vi "0 OCU - Networked.vi"() -> ()   [LabVIEW 2011]
doc: "This is the current implementation of the operator control unit (OCU) for small RC boat controlled by a host computer. The following features are currently implemented:\n- override control of the rudden angle and sail value by control interface or using keys\n- ability to add missions before and during a run\n- indicators for all relevant system status information\n\nAuthor: Jared Kirschner"
uses:
  2-Think/2 Typedefs/setpoints to boat.ctl
  2-Think/2 Typedefs/sail setpt.ctl
  2-Think/2 Typedefs/rudder angle.ctl
  2-Think/2 Typedefs/Velocity.ctl
  2-Think/2 Typedefs/apparent wind direction.ctl
  2-Think/2 Typedefs/apparent wind speed.ctl
  2-Think/2 Typedefs/apparent wind.ctl
  2-Think/2 Typedefs/heading.ctl
  2-Think/2 Typedefs/UTM Location.ctl
  2-Think/2 Typedefs/Which Boat.ctl
  2-Think/2 Typedefs/generalized sensor status.ctl
  2-Think/2 Typedefs/indicator LED.ctl
  2-Think/2 Typedefs/generalized actuator status.ctl
  0x2-OCU-Think Comm/0x2 Typedefs/Waypoints List.ctl
  0x2-OCU-Think Comm/0x2 Typedefs/ocuWaypoint.ctl
  0x2-OCU-Think Comm/0x2 Typedefs/waypointTypes.ctl
  0x2-OCU-Think Comm/0x2 Typedefs/Current Waypoint.ctl
  2-Think/2 Typedefs/robot velocity.ctl
  0x2-OCU-Think Comm/0x2 Typedefs/manual override.ctl
  0x2-OCU-Think Comm/0x2 Typedefs/ocuMessage.ctl
  0x2-OCU-Think Comm/0x2 Typedefs/ocuCommands.ctl
  2-Think/2 Typedefs/eStopCommand.ctl
  0x2-OCU-Think Comm/0x2 Typedefs/RIO-OCU update controls.ctl
  2-Think/2 Typedefs/rate of turn.ctl
  2-Think/2 Typedefs/pitch and roll.ctl
  2-Think/2 Typedefs/absolute wind direction.ctl
  2-Think/2 Typedefs/absolute wind speed.ctl
  2-Think/2 Typedefs/absolute water current vector.ctl
  0x2-OCU-Think Comm/0x2 Classes/NetworkStreams/Reader/readType.ctl
  2-Think/2 Globals/2 Global.vi
  0x2-OCU-Think Comm/0x2 Classes/NetworkStreams/Reader/NetworkStreamReader.lvclass
  0x2-OCU-Think Comm/0x2 Classes/NetworkStreams/Writer/NetworkStreamWriter.lvclass
panel:
  out "Rudder Position":dbl(knob) scale=50.0..-50.0 scale format="%#.2g"
  out "Sail Position":dbl(knob)
  out "Last update":timestamp
  out "Connected?":bool caption="Connection Status"
  in  "Location of THINK":string(combo)="127.0.0.1"
  in  "OVERRIDE SAIL?":bool
  in  "OVERRIDE RUDDER?":bool
  in  "E-Stop":bool
  out "Override Rudder Angle":dbl(slide) scale=-50.0..50.0
  out "Override Sail Value":dbl(slide) scale=0.0..1.0
  in  "OCU Tab Control":T1(tab)=enum."Before Mission: Define Mission"
  out "Connected":bool
  in  "Connect":bool
  out "Rudder Actuator Status":T2
  out "Sail Actuator Status":T2
  out "Wind Sensor Status":T4
  in  "Map Path (relative)":path=path "locations/LPB Pool.png"
  out "# of Waypts":i32
  in  "Save Waypoints\nand PoI":bool
  in  "Save Image":bool
  out "Mission Map":T5(plugin-control)
  in  "Delete Last Waypoint":bool
  in  "Mission Def Filepath":path caption="MDF (Mission Definition File) path (leave blank for nothing)"
  in  "Next Point Dist/Time":dbl=0.5
  in  "Next Point Type":T6
  in  "Globals":T7(tab)
  out "Which Boat Am I?":T8
  out "Battery Voltage":dbl
  out "Robot Heading":T9 format="%05.1f"
  out "Robot UTM Location":T10
  out "Overview Image":T5(plugin-control)
  out "Robot Velocity":T11
  out "Absolute Wind":T12
  out "Apparent Wind Direction":T13
  out "Apparent Wind Speed":T14
  out "Apparent Wind":T15
  out "Setpoints to boat":T16
  out "Sail Position":T17
  out "Rudder Angle":T18
  out "Waypoints Array":T19
  out "Current Waypoint":T21
  in  "Reset to start":bool
  out "Manual Override":T22
  # "TODO (Jason): finish this new representation"
  # "Manual Overide Control"
  # "Full Out = RIGHT"
  # "Out = UP"
  # "In = DOWN"
  # "Full In = LEFT"
  # "PORT"
  # "STARB"
  # "A"
  # "G"
  # "S"
  # "<--"
  # "D"
  # "-->"
  # "F"
  # "Map (required) and MDF (optional) are loaded on VI start.\nClick on map to add waypoints, pre-select attributes at right ->\nClick the appropriate buttons to save MDFs."
  # "As Measured"
  # "From Planning Functions"
  # "Path Planning"
  # "(this is not a cluster because subitems\nare generated in parallel code)"
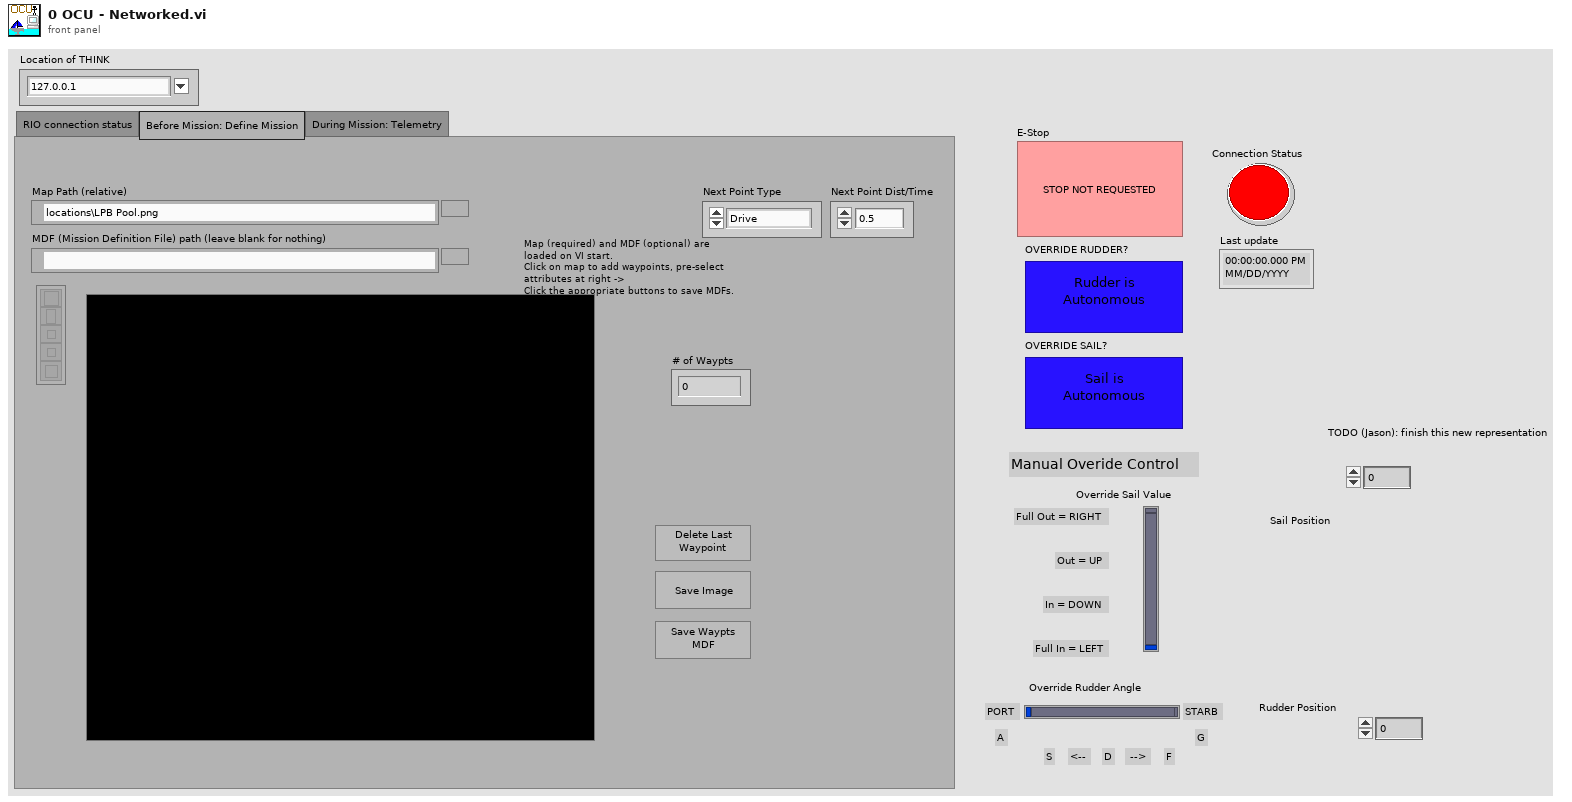
[diagram p1: front panel]
types:
  T1 = enum32{"RIO connection status", "Before Mission: Define Mission", "During Mission: Telemetry"}
  T2 = typedef "generalized actuator status.ctl" = cluster{"Actuator Connected":T3}
  T3 = typedef "indicator LED.ctl" = bool
  T4 = typedef "generalized sensor status.ctl" = cluster{"Sensor Connected":T3, "Sensor Initialized":T3, "Sensor OK":T3, "Latest Error String":string, "GPS Lock":T3}
  T5 = typedef "IMAQ Image.ctl" = refnum<image>
  T6 = typedef "waypointTypes.ctl" = enum16{"Drive", "Round Port", "Round Starboard", "Stay"}
  T7 = enum32{"How Am I", "Where Am I", "What's Around Me", "Path Planning"}
  T8 = typedef "Which Boat.ctl" = enum16{"Competition Boat", "Small RC", "Simulation"}
  T9 = typedef "heading.ctl" = dbl
  T10 = typedef "UTM Location.ctl" = cluster{"UTM Zone":dbl, "Hemisphere":enum16{"North", "South"}, "East":dbl, "North":dbl}
  T11 = typedef "robot velocity.ctl" = cluster{"East":dbl, "North":dbl}
  T12 = typedef "Velocity.ctl" = cluster{"East":dbl, "North":dbl}
  T13 = typedef "apparent wind direction.ctl" = dbl
  T14 = typedef "apparent wind speed.ctl" = dbl
  T15 = typedef "apparent wind.ctl" = cluster{"Toward Fore":dbl, "Toward Starboard":dbl}
  T16 = typedef "setpoints to boat.ctl" = cluster{"Sail Position":T17, "Rudder Angle":T18}
  T17 = typedef "sail setpt.ctl" = dbl
  T18 = typedef "rudder angle.ctl" = dbl
  T19 = typedef "Waypoints List.ctl" = T20[]
  T20 = typedef "ocuWaypoint.ctl" = cluster{"Point Type":T6, "Dist/Time":dbl, "UTM Location":T10}
  T21 = typedef "Current Waypoint.ctl" = i32
  T22 = typedef "manual override.ctl" = cluster{"Override Active Rudder":bool, "Setpoints":T16, "Override Active Sail":bool}
  T23 = typedef "RIO-OCU update controls.ctl" = cluster{"Sensor Status":T4, "Battery Voltage":dbl, "Rudder Actuator Status":T2, "Sail Actuator Status":T2, "Which Boat Am I?":T8, "Robot Velocity":T11, "Robot UTM Location":T10, "Robot\nHeading ":T9, "Robot\nRate of Turn":T24, "Robot Pitch/Roll":T25, "Apparent Wind":T15, "Apparent Wind\nSpeed":T14, "Apparent Wind\nDirection (º)":T13, "Absolute Wind":T12, "Absolute Wind\nDirection (º)":T26, "Absolute Wind\nSpeed":T27, "Absolute Water Current Vector":T28, "Rudder Angle":T18, "Sail Position":T17, "Manual Override Cluster":T22, "Setpoints to boat":T16, "Waypoints Array":T19, "Current Waypoint":T21, "Think freq.":dbl, "Sense freq.":dbl, "Act freq.":dbl, "E-stop freq.":dbl, "Network \nfreq.":dbl, "Network \nLoop Iterations":i64, "E-Stop":bool}
  T24 = typedef "rate of turn.ctl" = dbl
  T25 = typedef "pitch and roll.ctl" = cluster{"Pitch":dbl, "Roll":dbl}
  T26 = typedef "absolute wind direction.ctl" = dbl
  T27 = typedef "absolute wind speed.ctl" = dbl
  T28 = typedef "absolute water current vector.ctl" = cluster{"Direction":T13, "Magnitude":T13}
  T29 = typedef "ocuMessage.ctl" = cluster{"OCU Command":T30, "Data":variant}
  T30 = typedef "ocuCommands.ctl" = enum16{"Pass", "Send override", "Add waypoints", "Delete waypoint", "Set waypoint number", "Stop"}
  T31 = typedef "0-Image Descriptor.ctl" = cluster{"Upper-Left Corner Coordinates":T10, "Meters/Pixel":dbl}
  T32 = typedef "eStopCommand.ctl" = enum16{"Reset E-Stop", "Get E-Stop", "Set E-Stop"}
  T33 = typedef "eventvkey.ctl" = enum16{"ASCII", "Enter", "Return", "Shift", "Ctrl", "Alt", "Cmd", "Opt", "Caps", "NumLock", "Clear", "Break", "Up", "Down", "Left", "Right", "Insert", "Delete", "Home", "End", "PageUp", "PageDown", "Escape", "Help", "Pause", "ScrollLock", "F1", "F2", "F3", "F4", "F5", "F6", "F7", "F8", "F9", "F10", "F11", "F12", "F13", "F14", "F15", "F16", "F17", "F18", "F19", "F20", "F21", "F22", "F23", "F24", "Play", "VolumeUp", "VolumeDown", "Mute", "Two Byte Char"}
  T34 = typedef "NetworkStreamReader.lvclass/readType.ctl" = enum16{"Next in buffer", "Most current"}
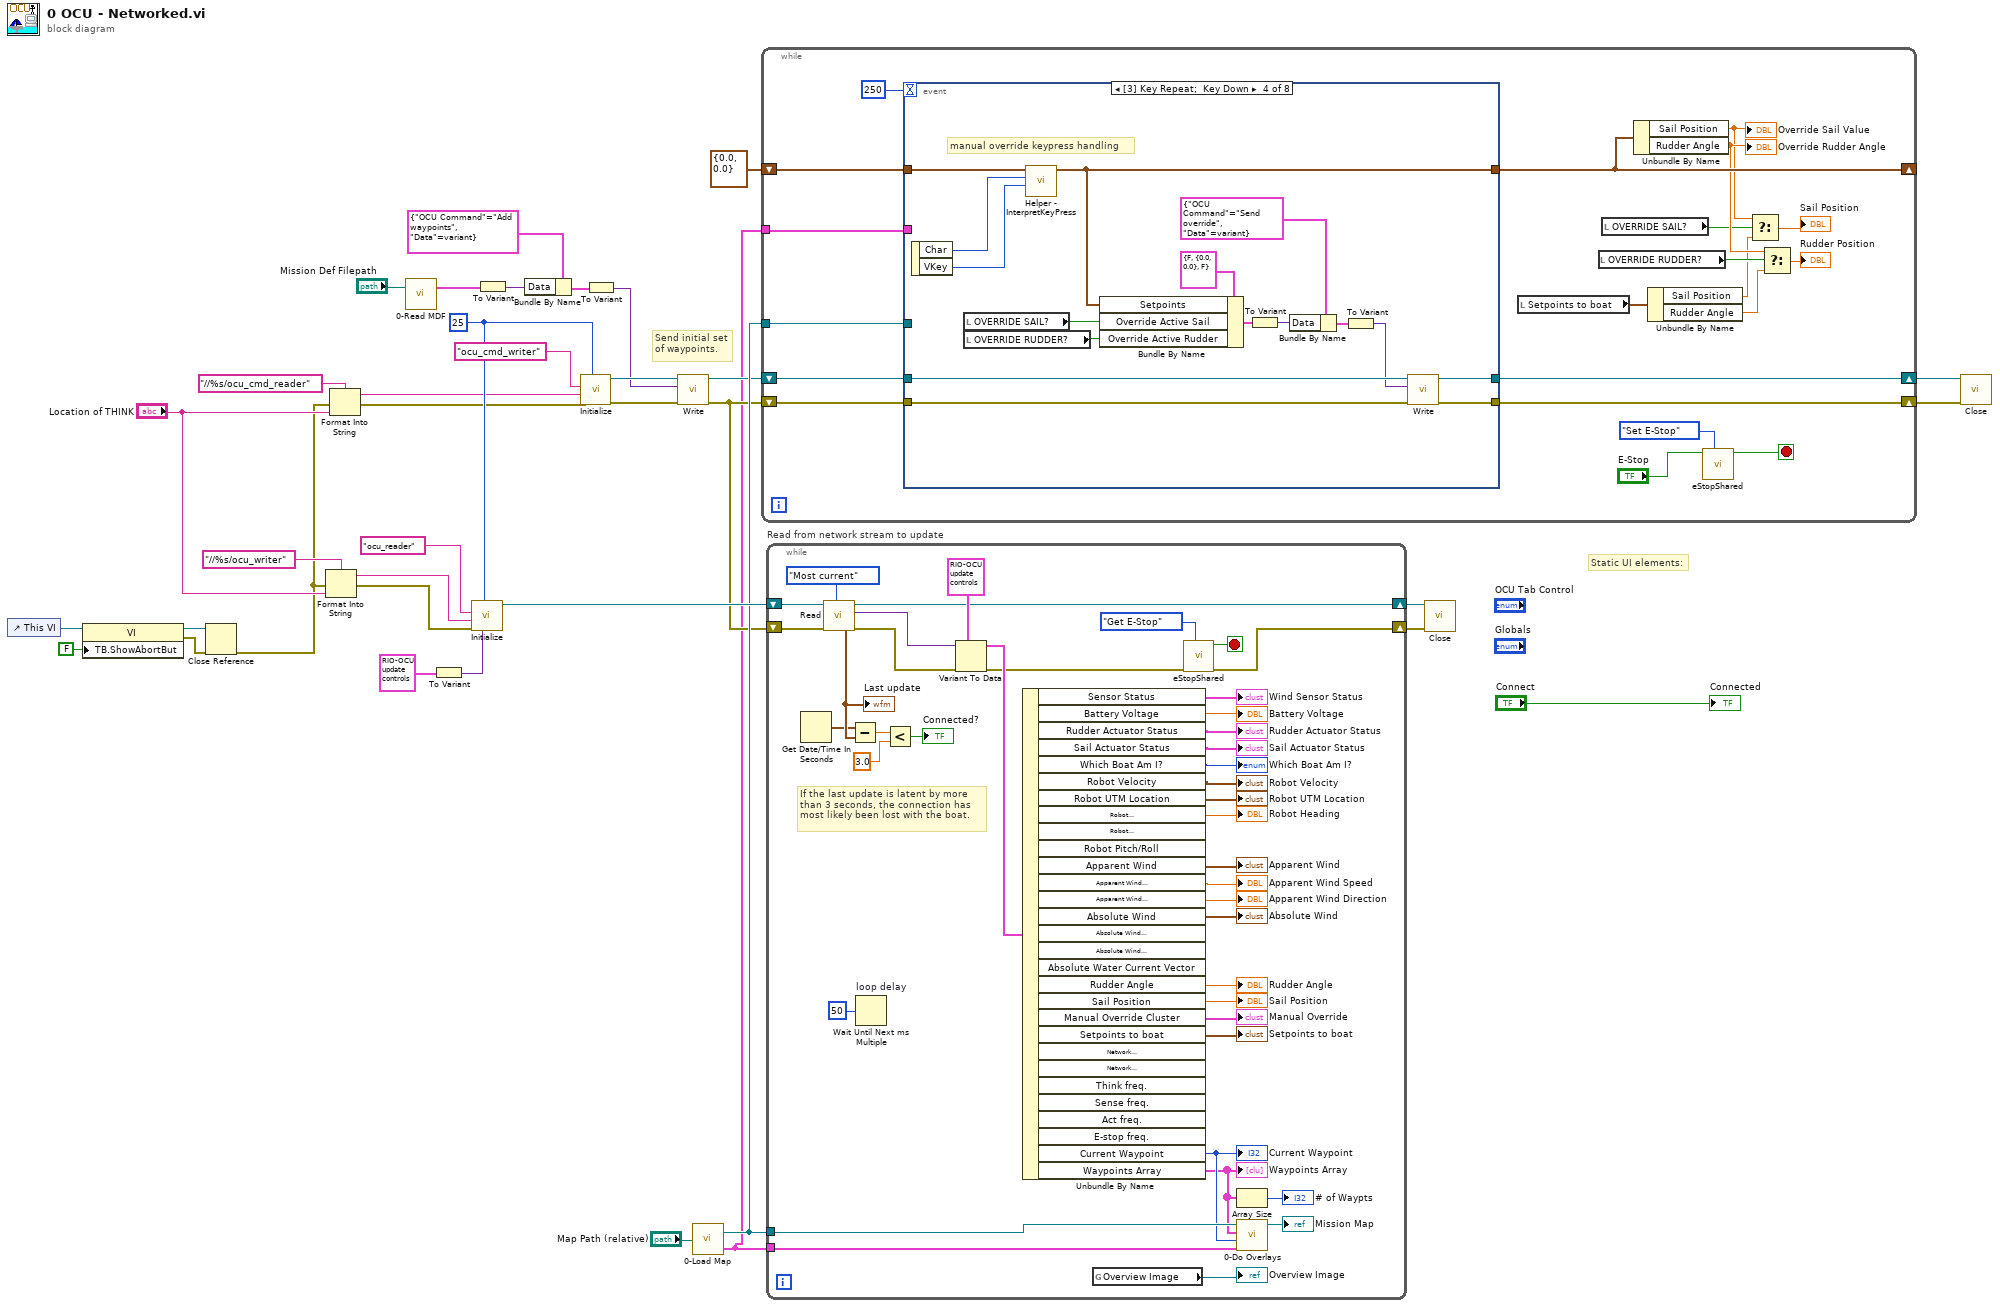
[diagram p0: block diagram]
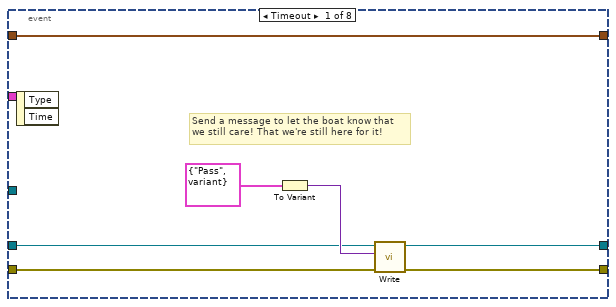
[diagram p2: hidden frame]
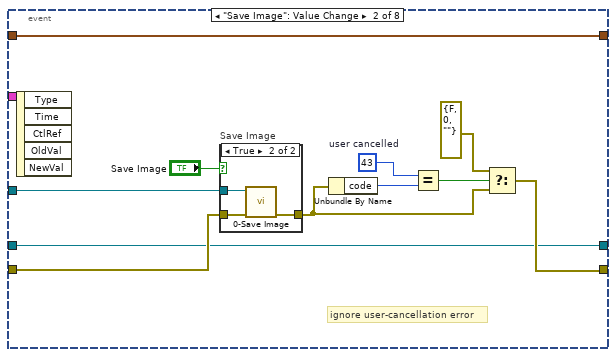
[diagram p3: hidden frame]
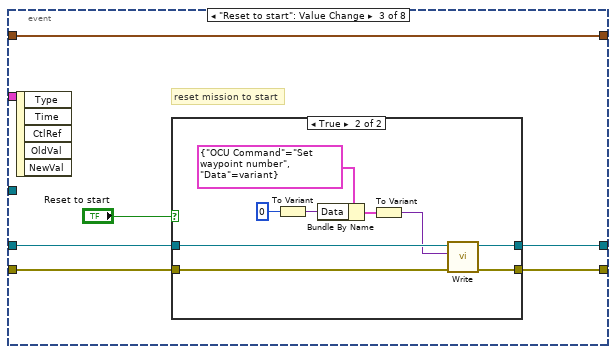
[diagram p5: hidden frame]
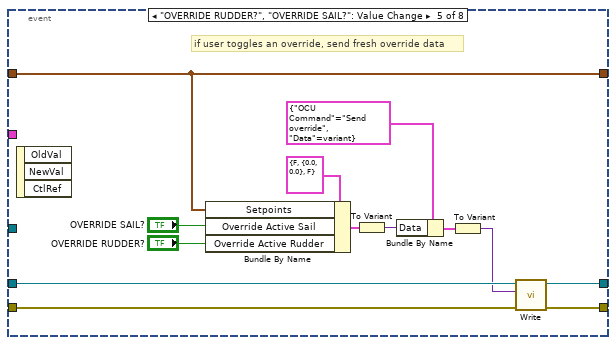
[diagram p7: hidden frame]
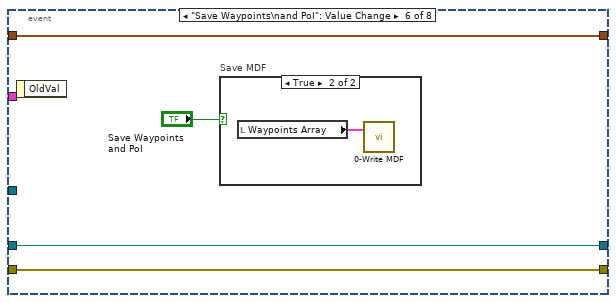
[diagram p8: hidden frame]
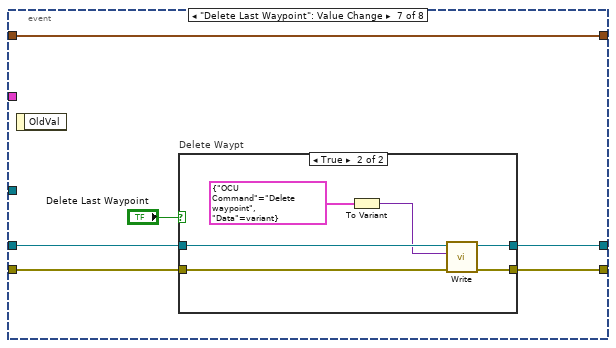
[diagram p10: hidden frame]
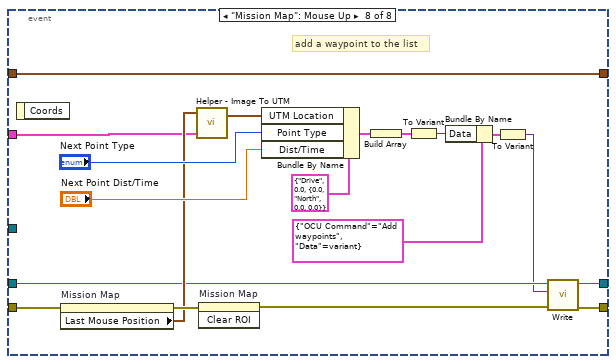
[diagram p12: hidden frame]
diagram:
  w31 = 25 ("writer buffer size")
  # "Send initial set\nof waypoints."
  # "Static UI elements:"
  n1 = control-ref of="This VI"() -> (w9:refnum<vi>)
  n2 = property class="VI"(reference=w9, "TB.ShowAbortBut"=FALSE ("Tool Bar:Show Abort Button")) -> (reference out=w7:refnum<vi>, error out=w6:errorcluster)  [unwired: 1 in]
  n3 = Close Reference(reference=w7, error in (no error)=w6) -> (error out=w5:errorcluster)
  n4 = Format Into String(format string="//%s/ocu_writer", error in=w5, "Location of THINK") -> (resulting string=w15:string, error out=w3:errorcluster)  [unwired: 1 in]
  n5 = Format Into String(format string="//%s/ocu_cmd_reader", error in=w5, "Location of THINK") -> (resulting string=w13:string, error out=w4:errorcluster)  [unwired: 1 in]
  n6 = call "0-Read MDF.vi"("MDF file path"="Mission Def Filepath") -> ("Waypoints List"=w17:T19)  [unwired: 1 in, 1 out]
  n7 = To Variant(anything=T23 {"Sensor Status"={"Sensor Connected"=FALSE, "Sensor Initialized"=FALSE, "Sensor OK"=FALSE, "Latest Error String"="", "GPS Lock"=FALSE}, "Battery Voltage"=0.0, "Rudder Actuator Status"={"Actuator Connected"=FALSE}, "Sail Actuator Status"={"Actuator Connected"=FALSE}, "Which Boat Am I?"=enum."Competition Boat", "Robot Velocity"={"East"=0.0, "North"=0.0}, "Robot UTM Location"={"UTM Zone"=0.0, "Hemisphere"=enum."North", "East"=0.0, "North"=0.0}, "Robot\nHeading "=0.0, "Robot\nRate of Turn"=0.0, "Robot Pitch/Roll"={"Pitch"=0.0, "Roll"=0.0}, "Apparent Wind"={"Toward Fore"=0.0, "Toward Starboard"=0.0}, "Apparent Wind\nSpeed"=0.0, "Apparent Wind\nDirection (º)"=0.0, "Absolute Wind"={"East"=0.0, "North"=0.0}, "Absolute Wind\nDirection (º)"=0.0, "Absolute Wind\nSpeed"=0.0, "Absolute Water Current Vector"={"Direction"=0.0, "Magnitude"=0.0}, "Rudder Angle"=0.0, "Sail Position"=0.0, "Manual Override Cluster"={"Override Active Rudder"=FALSE, "Setpoints"={"Sail Position"=0.0, "Rudder Angle"=0.0}, "Override Active Sail"=FALSE}, "Setpoints to boat"={"Sail Position"=0.0, "Rudder Angle"=0.0}, "Waypoints Array"=[], "Current Waypoint"=0, "Think freq."=0.0, "Sense freq."=0.0, "Act freq."=0.0, "E-stop freq."=0.0, "Network \nfreq."=0.0, "Network \nLoop Iterations"=0, "E-Stop"=FALSE} ("RIO->OCU update data")) -> (Variant=w30:variant)
  n8 = call "Initialize.vi"("Default return"=w30, "writer buffer size"=w31, "error in (no error)"=w3, "writer url"=w15, "reader name"="ocu_reader" ("writer name")) -> ("NetworkStreamWriter out"=w33:refnum<class "NetworkStreamReader.lvclass">)  [unwired: 5 in, 1 out]
  n9 = To Variant(anything=w17) -> (Variant=w18:variant)
  n10 = Bundle By Name(cluster=T29 {"OCU Command"=enum."Add waypoints", "Data"=variant}, "Data"=w18) -> (w20:T29)
  n11 = call "Initialize.vi"("writer buffer size"=w31, "error in (no error)"=w4, "reader url"=w13, "writer name"="ocu_cmd_writer") -> ("error out"=w24:errorcluster, "NetworkStreamWriter out"=w25:refnum<class "NetworkStreamWriter.lvclass">)  [unwired: 6 in]
  n12 = To Variant(anything=w20) -> (Variant=w19:variant)
  n13 = call "Write.vi"("error in (no error)"=w24, "element"=w19, "NetworkStreamWriter in"=w25) -> ("error out"=w23:errorcluster, "NetworkStreamWriter out"=w22:refnum<class "NetworkStreamWriter.lvclass">)  [unwired: 7 in]
  n14 = call "0-Load Map.vi"("Image Path"="Map Path (relative)") -> ("Image Out"=w26:T5, "Image Descriptor"=w1:T31)
  n15 = while {
    shift-right: [w56] -> w10
    shift-left: w23 -> [w52]
    shift-right: [w48] -> _
    shift-left: T16 {"Sail Position"=0.0, "Rudder Angle"=0.0} ("Setpoints") -> [w58]
    shift-right: [w50] -> w11
    shift-left: w22 -> [w51]
    tunnel: w26 -> [w49]
    tunnel: w1 -> [w47]
    stop <- w55 stop-if-true
    n16 = event shown="[3] Key Repeat;  Key Down" {
      selector: _ -> [_ _ _ _ _ _ _ _]
      dyn-events: _ -> [_ _ _ _ _ _ _ _]
      timeout: 250 -> [_ _ _ _ _ _ _ _]
      tunnel: w58 -> [w65 w72 w86 w113 w116 w129 w136 w160]
      tunnel: [w65 w72 w86 w109 w116 w129 w136 w160] -> w48
      tunnel: w52 -> [w59 w70 w83 w106 w123 w128 w134 w157]
      tunnel: [w60 w67 w81 w105 w122 w128 w132 w150] -> w56
      tunnel: w51 -> [w62 w66 w84 w108 w125 w127 w135 w152]
      tunnel: [w61 w66 w82 w107 w124 w127 w133 w151] -> w50
      tunnel: w49 -> [_ w71 _ _ _ _ _ _]
      tunnel: w47 -> [_ _ _ _ _ _ _ w146]
      event Timeout {
        # "Send a message to let the boat know that\nwe still care! That we're still here for it!"
        n17 = event-data() -> ()  [unwired: 1 in, 2 out]
        n18 = To Variant(anything=T29 {"OCU Command"=enum."Pass", "Data"=variant}) -> (Variant=w63:variant)
        n19 = call "Write.vi"("error in (no error)"=w59, "element"=w63, "NetworkStreamWriter in"=w62) -> ("error out"=w60:errorcluster, "NetworkStreamWriter out"=w61:refnum<class "NetworkStreamWriter.lvclass">)  [unwired: 7 in]
      }
      event "Save Image": Value Change {
        w75 = 43  # user cancelled
        # "ignore user-cancellation error"
        n20 = event-data() -> ()  [unwired: 1 in, 5 out]
        n21 = case "Save Image" shown="True" "Save Image" {
          tunnel: w70 -> [w77 w80]
          tunnel: [w77 w79] -> w69
          tunnel: w71 -> [_ w78]
          frame False {
          }
          frame True {
            n22 = call "0-Save Image.vi"("Error In"=w80, "Image in"=w78) -> ("Error Out"=w79:errorcluster)  [unwired: 9 in]
          }
        }
        n23 = Unbundle By Name(w69) -> ("code"=w76:i32)
        n24 = Equal?(x=w75, y=w76) -> (x = y?=w74:bool)
        n25 = Select(t=errorcluster {"status"=FALSE, "code"=0, "source"=""}, s=w74, f=w69) -> (s? t:f=w67:errorcluster)
      }
      event "Reset to start": Value Change {
        # "reset mission to start"
        n26 = event-data() -> ()  [unwired: 1 in, 5 out]
        n27 = case shown="True" "Reset to start" {
          tunnel: w84 -> [w88 w94]
          tunnel: w83 -> [w87 w95]
          tunnel: [w88 w97] -> w82
          tunnel: [w87 w96] -> w81
          frame False {
          }
          frame True {
            n28 = To Variant(anything=T21 0 ("Current Waypoint")) -> (Variant=w92:variant)
            n29 = Bundle By Name(cluster=T29 {"OCU Command"=enum."Set waypoint number", "Data"=variant}, "Data"=w92) -> (w90:T29)
            n30 = To Variant(anything=w90) -> (Variant=w89:variant)
            n31 = call "Write.vi"("error in (no error)"=w95, "element"=w89, "NetworkStreamWriter in"=w94) -> ("error out"=w96:errorcluster, "NetworkStreamWriter out"=w97:refnum<class "NetworkStreamWriter.lvclass">)  [unwired: 7 in]
          }
        }
      }
      event Key Repeat; Key Down {
        # "manual override keypress handling"
        n32 = event-data() -> ("Char"=w112:i16, "VKey"=w111:T33)  [unwired: 1 in]
        n33 = local read "OVERRIDE SAIL?"() -> (w98:bool)
        n34 = local read "OVERRIDE RUDDER?"() -> (w99:bool)
        n35 = call "Helper - InterpretKeyPress.vi"("VKey"=w111, "Char"=w112, "Command In"=w113) -> ("Command Out"=w109:T16)  [unwired: 8 in]
        n36 = Bundle By Name(cluster=T22 {"Override Active Rudder"=FALSE, "Setpoints"={"Sail Position"=0.0, "Rudder Angle"=0.0}, "Override Active Sail"=FALSE} ("Manual Override Cluster"), "Setpoints"=w109, "Override Active Sail"=w98, "Override Active Rudder"=w99) -> (w101:T22)
        n37 = To Variant(anything=w101) -> (Variant=w104:variant)
        n38 = Bundle By Name(cluster=T29 {"OCU Command"=enum."Send override", "Data"=variant}, "Data"=w104) -> (w103:T29)
        n39 = To Variant(anything=w103) -> (Variant=w100:variant)
        n40 = call "Write.vi"("error in (no error)"=w106, "element"=w100, "NetworkStreamWriter in"=w108) -> ("error out"=w105:errorcluster, "NetworkStreamWriter out"=w107:refnum<class "NetworkStreamWriter.lvclass">)  [unwired: 7 in]
      }
      event "OVERRIDE RUDDER?", "OVERRIDE SAIL?": Value Change {
        # "if user toggles an override, send fresh override data"
        n41 = event-data() -> ()  [unwired: 1 in, 3 out]
        n42 = Bundle By Name(cluster=T22 {"Override Active Rudder"=FALSE, "Setpoints"={"Sail Position"=0.0, "Rudder Angle"=0.0}, "Override Active Sail"=FALSE} ("Manual Override Cluster"), "Setpoints"=w116, "Override Active Sail"="OVERRIDE SAIL?", "Override Active Rudder"="OVERRIDE RUDDER?") -> (w118:T22)
        n43 = To Variant(anything=w118) -> (Variant=w121:variant)
        n44 = Bundle By Name(cluster=T29 {"OCU Command"=enum."Send override", "Data"=variant}, "Data"=w121) -> (w120:T29)
        n45 = To Variant(anything=w120) -> (Variant=w117:variant)
        n46 = call "Write.vi"("error in (no error)"=w123, "element"=w117, "NetworkStreamWriter in"=w125) -> ("error out"=w122:errorcluster, "NetworkStreamWriter out"=w124:refnum<class "NetworkStreamWriter.lvclass">)  [unwired: 7 in]
      }
      event "Save Waypoints\nand PoI": Value Change {
        n47 = event-data() -> ()  [unwired: 1 in, 1 out]
        n48 = case "Save MDF" shown="True" "Save Waypoints\nand PoI" {
          frame False {
          }
          frame True {
            n49 = local read "Waypoints Array"() -> (w131:T19)
            n50 = call "0-Write MDF.vi"("Waypoints List"=w131) -> ()  [unwired: 2 in, 1 out]
          }
        }
      }
      event "Delete Last Waypoint": Value Change {
        n51 = event-data() -> ()  [unwired: 1 in, 1 out]
        n52 = case "Delete Waypt" shown="True" "Delete Last Waypoint" {
          tunnel: w135 -> [w139 w145]
          tunnel: w134 -> [w138 w144]
          tunnel: [w139 w143] -> w133
          tunnel: [w138 w142] -> w132
          frame False {
          }
          frame True {
            n53 = To Variant(anything=T29 {"OCU Command"=enum."Delete waypoint", "Data"=variant}) -> (Variant=w140:variant)
            n54 = call "Write.vi"("error in (no error)"=w144, "element"=w140, "NetworkStreamWriter in"=w145) -> ("error out"=w142:errorcluster, "NetworkStreamWriter out"=w143:refnum<class "NetworkStreamWriter.lvclass">)  [unwired: 7 in]
          }
        }
      }
      event "Mission Map": Mouse Up {
        # "add a waypoint to the list"
        n55 = event-data() -> ()  [unwired: 1 in, 1 out]
        n56 = property on="Mission Map" class="ImageControl"(error in=w157) -> (error out=w159:errorcluster, "Last Mouse Position"=w158:cluster{"X":i32, "Y":i32})  [unwired: 1 in, 1 out]
        n57 = call "Helper - Image To UTM.vi"("Image Descriptor"=w146, "Pixel Coordinates"=w158) -> ("UTM Location"=w162:T10)  [unwired: 1 in, 1 out]
        n58 = invoke on="Mission Map" class="ImageControl" method="Clear ROI"(error in=w159) -> (error out=w149:errorcluster)  [unwired: 2 in, 2 out]
        n59 = Bundle By Name(cluster=T20 {"Point Type"=enum."Drive", "Dist/Time"=0.0, "UTM Location"={"UTM Zone"=0.0, "Hemisphere"=enum."North", "East"=0.0, "North"=0.0}} ("Waypoint 2"), "UTM Location"=w162, "Point Type"="Next Point Type", "Dist/Time"="Next Point Dist/Time") -> (w156:T20)
        n60 = Build Array(w156) -> (w154:T20[])
        n61 = To Variant(anything=w154) -> (Variant=w153:variant)
        n62 = Bundle By Name(cluster=T29 {"OCU Command"=enum."Add waypoints", "Data"=variant}, "Data"=w153) -> (w148:T29)
        n63 = To Variant(anything=w148) -> (Variant=w147:variant)
        n64 = call "Write.vi"("error in (no error)"=w149, "element"=w147, "NetworkStreamWriter in"=w152) -> ("error out"=w150:errorcluster, "NetworkStreamWriter out"=w151:refnum<class "NetworkStreamWriter.lvclass">)  [unwired: 7 in]
      }
    }
    n65 = local read "Setpoints to boat"() -> (w40:T16)
    n66 = local read "OVERRIDE RUDDER?"() -> (w46:bool)
    n67 = local read "OVERRIDE SAIL?"() -> (w41:bool)
    n68 = Unbundle By Name(w48) -> ("Sail Position"=w43:T17, "Rudder Angle"=w44:T18)
    "Override Sail Value" <- w43
    "Override Rudder Angle" <- w44
    n69 = Unbundle By Name(w40) -> ("Sail Position"=w39:T17, "Rudder Angle"=w38:T18)
    n70 = call "eStopShared.vi"("Command"=eStopCommand."Set E-Stop", "E-Stop"="E-Stop") -> ("E-Stop Out"=w55:bool)  [unwired: 8 in, 1 out]
    n71 = Select(t=w43, s=w41, f=w39) -> (s? t:f=→"Sail Position":T17)
    n72 = Select(t=w44, s=w46, f=w38) -> (s? t:f=→"Rudder Position":T18)
  }
  n73 = while "Read from network stream to update" {
    shift-right: [w199] -> w28
    shift-left: w33 -> [w205]
    shift-right: [w198] -> w27
    shift-left: w23 -> [w204]
    tunnel: w26 -> [w176]
    tunnel: w1 -> [w177]
    stop <- w196 stop-if-true
    # "If the last update is latent by more\nthan 3 seconds, the connection has\nmost likely been lost with the boat."
    n74 = Get Date/Time In Seconds() -> (seconds since 1Jan1904=w168:timestamp)
    n75 = call "Read.vi"("Read Type"=readType."Most current", "error in (no error)"=w204, "NetworkStreamReader in"=w205) -> ("error out"=w202:errorcluster, "element"=w201:variant, "NetworkStreamReader out"=w199:refnum<class "NetworkStreamReader.lvclass">, "Time Stamp"=w169:timestamp)  [unwired: 4 in, 1 out]
    "Last update" <- w169
    n76 = Subtract(x=w168, y=w169) -> (x-y=w167:dbl)
    n77 = Wait Until Next ms Multiple "loop delay"(millisecond multiple=u32 50) -> ()  [unwired: 1 out]
    n78 = Less?(x=w167, y=3.0) -> (x < y?=→"Connected?":bool)
    n79 = Variant To Data(error in=w202, type=T23 {"Sensor Status"={"Sensor Connected"=FALSE, "Sensor Initialized"=FALSE, "Sensor OK"=FALSE, "Latest Error String"="", "GPS Lock"=FALSE}, "Battery Voltage"=0.0, "Rudder Actuator Status"={"Actuator Connected"=FALSE}, "Sail Actuator Status"={"Actuator Connected"=FALSE}, "Which Boat Am I?"=enum."Competition Boat", "Robot Velocity"={"East"=0.0, "North"=0.0}, "Robot UTM Location"={"UTM Zone"=0.0, "Hemisphere"=enum."North", "East"=0.0, "North"=0.0}, "Robot\nHeading "=0.0, "Robot\nRate of Turn"=0.0, "Robot Pitch/Roll"={"Pitch"=0.0, "Roll"=0.0}, "Apparent Wind"={"Toward Fore"=0.0, "Toward Starboard"=0.0}, "Apparent Wind\nSpeed"=0.0, "Apparent Wind\nDirection (º)"=0.0, "Absolute Wind"={"East"=0.0, "North"=0.0}, "Absolute Wind\nDirection (º)"=0.0, "Absolute Wind\nSpeed"=0.0, "Absolute Water Current Vector"={"Direction"=0.0, "Magnitude"=0.0}, "Rudder Angle"=0.0, "Sail Position"=0.0, "Manual Override Cluster"={"Override Active Rudder"=FALSE, "Setpoints"={"Sail Position"=0.0, "Rudder Angle"=0.0}, "Override Active Sail"=FALSE}, "Setpoints to boat"={"Sail Position"=0.0, "Rudder Angle"=0.0}, "Waypoints Array"=[], "Current Waypoint"=0, "Think freq."=0.0, "Sense freq."=0.0, "Act freq."=0.0, "E-stop freq."=0.0, "Network \nfreq."=0.0, "Network \nLoop Iterations"=0, "E-Stop"=FALSE} ("RIO->OCU update data"), Variant=w201) -> (data=w195:T23, error out=w171:errorcluster)
    n80 = Unbundle By Name(w195) -> ("Sensor Status"=→"Wind Sensor Status":T4, "Battery Voltage"=→"Battery Voltage":dbl, "Rudder Actuator Status"=→"Rudder Actuator Status":T2, "Sail Actuator Status"=→"Sail Actuator Status":T2, "Which Boat Am I?"=→"Which Boat Am I?":T8, "Robot Velocity"=→"Robot Velocity":T11, "Robot UTM Location"=→"Robot UTM Location":T10, "Robot\nHeading"=→"Robot Heading":T9, "Apparent Wind"=→"Apparent Wind":T15, "Apparent Wind\nSpeed"=→"Apparent Wind Speed":T14, "Apparent Wind\nDirection (º)"=→"Apparent Wind Direction":T13, "Absolute Wind"=→"Absolute Wind":T12, "Rudder Angle"=→"Rudder Angle":T18, "Sail Position"=→"Sail Position":T17, "Manual Override Cluster"=→"Manual Override":T22, "Setpoints to boat"=→"Setpoints to boat":T16, "Current Waypoint"=w175:T21, "Waypoints Array"=w174:T19)  [unwired: 11 out]
    "Current Waypoint" <- w175
    "Waypoints Array" <- w174
    n81 = global read "2 Global.vi" "Overview Image"() -> (→"Overview Image":T5)
    n82 = call "eStopShared.vi"("Command"=eStopCommand."Get E-Stop", "Error In"=w171) -> ("Error Out"=w198:errorcluster, "E-Stop Out"=w196:bool)  [unwired: 8 in]
    n83 = Array Size(array=w174) -> (size(s)=→"# of Waypts":i32)
    n84 = call "0-Do Overlays.vi"("Image Descriptor"=w177, "Current Waypoint #"=w175, "Waypoints List"=w174, "Image in"=w176) -> ("Image out"=→"Mission Map":T5)  [unwired: 7 in]
  }
  n85 = call "Close.vi"("error in (no error)"=w27, "NetworkStreamReader in"=w28) -> ()  [unwired: 8 in, 2 out]
  n86 = call "Close.vi"("error in (no error)"=w10, "NetworkStreamWriter in"=w11) -> ()  [unwired: 8 in, 2 out]
  "Connected" <- "Connect"
